vi "X Listbox Facade.vi"(0 "Data In":T4, 2 "Display State In":T2, 3 "Container State":T3) -> (6 "Data Out":T4, 7 "Display State Out":T2, 8 "Action":T1)   [LabVIEW 2011, in "X Listbox-Solution.xctl"]
doc: "This is the facade for the X Listbox. Details about implementation can be found in the course manual.\n\nAAL 9/09"
uses:
  X Listbox-Solution.xctl
  X Listbox Data.ctl
  <vilib>/_xctls/Container State.ctl
  X Listbox State.ctl
  <vilib>/_xctls/Action.ctl
  <vilib>/_xctls/XControlSupport.lvlib
panel:
  in  "True Boolean":bool=TRUE
  in  "False Boolean":bool
  in  "Listbox":i32(listbox)
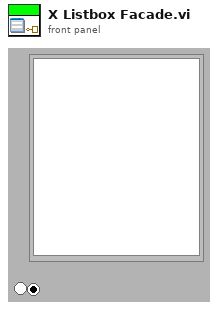
[diagram p1: front panel]
types:
  T1 = typedef "XControlSupport.lvlib/Action.ctl" = cluster{"Data Changed?":bool, "State Changed?":bool, "Action Name":string}
  T2 = typedef "X Listbox-Solution.xctl/X Listbox State.ctl" = cluster{"# Items":i32, "Names":string[]}
  T3 = typedef "XControlSupport.lvlib/Container State.ctl" = cluster{"Indicator?":bool, "Run Mode?":bool, " Refnum":refnum<vi>}
  T4 = typedef "X Listbox-Solution.xctl/X Listbox Data.ctl" = string
  T5 = typedef "imagedata.ctl" = cluster{"image type":i32, "image depth":i32, "image":u8[], "mask":u8[], "colors":u32[], "Rectangle":cluster{"left":i16, "top":i16, "right":i16, "bottom":i16}}
  T6 = typedef "LVPoint32TypeDef.ctl" = cluster{"Horizontal":i32, "Vertical":i32}
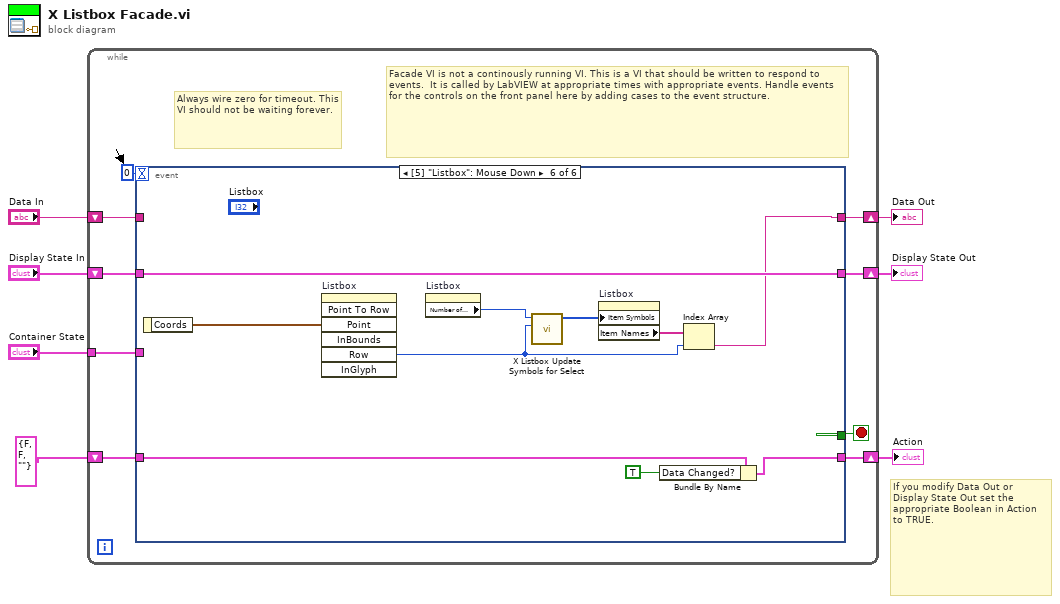
[diagram p0: block diagram]
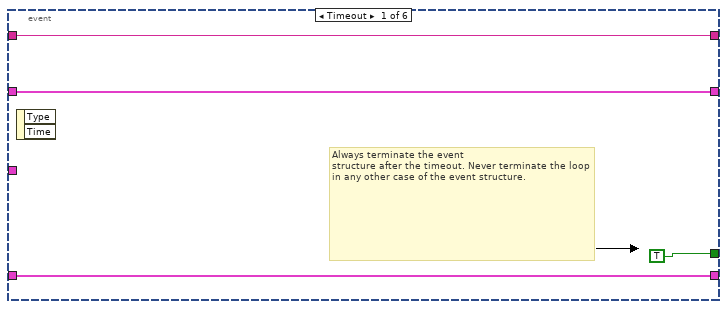
[diagram p2: hidden frame]
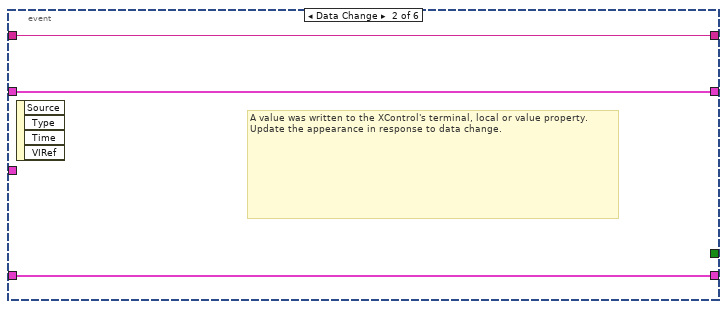
[diagram p3: hidden frame]
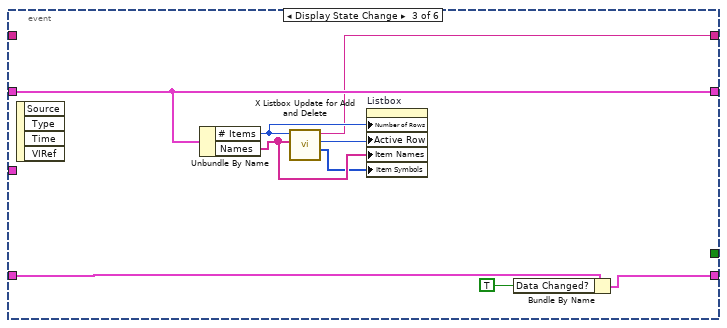
[diagram p4: hidden frame]
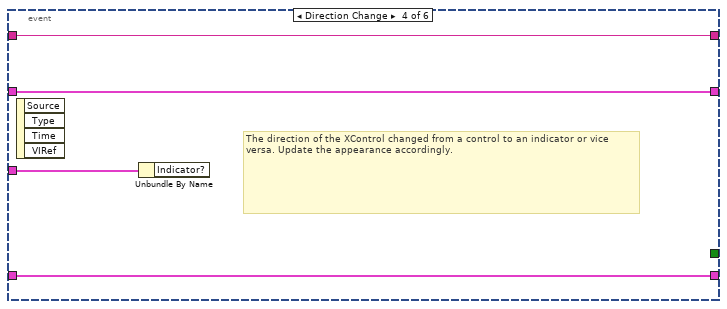
[diagram p5: hidden frame]
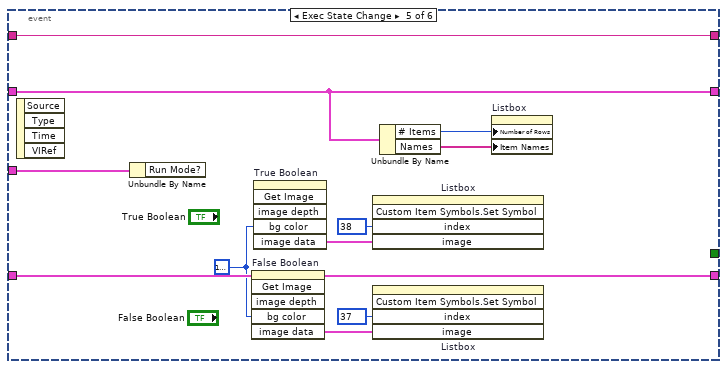
[diagram p6: hidden frame]
diagram:
  # "If you modify Data Out or\nDisplay State Out set the\nappropriate Boolean in Action\nto TRUE."
  n1 = while {
    shift-right: [w15] -> w4
    shift-left: "Display State In" -> [w16]
    tunnel: "Container State" -> [w12]
    shift-right: [w10] -> w7
    shift-left: "Data In" -> [w11]
    shift-right: [w8] -> w2
    shift-left: T1 {"Data Changed?"=FALSE, "State Changed?"=FALSE, "Action Name"=""} ("Action") -> [w9]
    stop <- w14 stop-if-true
    # "Facade VI is not a continously running VI. This is a VI that should be written to respond to events.  It is called by LabVIEW at appropriate times with appropriate events. Handle events for the controls on the front panel here by adding cases to the event structure."
    # "Always wire zero for timeout. This\nVI should not be waiting forever."
    n2 = event shown="[5] \"Listbox\": Mouse Down" {
      selector: _ -> [_ _ _ _ _ _]
      dyn-events: _ -> [_ _ _ _ _ _]
      timeout: 0 -> [_ _ _ _ _ _]
      tunnel: w16 -> [w18 w22 w32 w35 w44 w56]
      tunnel: [w18 w22 w32 w35 w44 w56] -> w15
      tunnel: [TRUE _ _ _ _ _] -> w14
      tunnel: w12 -> [_ _ _ w36 w47 _]
      tunnel: w11 -> [w17 w23 _ w34 w46 _]
      tunnel: [w17 w23 w30 w34 w46 w51] -> w10
      tunnel: [w19 w21 w25 w33 w45 w49] -> w8
      tunnel: w9 -> [w19 w21 w26 w33 w45 w50]
      event Timeout {
        # "Always terminate the event\nstructure after the timeout. Never terminate the loop in any other case of the event structure."
        n3 = event-data() -> ()  [unwired: 1 in, 2 out]
      }
      event Data Change {
        # "A value was written to the XControl's terminal, local or value property.\nUpdate the appearance in response to data change."
        n4 = event-data() -> ()  [unwired: 1 in, 4 out]
      }
      event Display State Change {
        n5 = event-data() -> ()  [unwired: 1 in, 4 out]
        n6 = Unbundle By Name(w32) -> ("# Items"=w31:i32, "Names"=w28:string[])
        n7 = call "X Listbox Update for Add and Delete.vi"("Names"=w28, "# Items"=w31) -> ("Item Symbols"=w27:i32[], "Active Row"=w29:i32, "Name"=w30:string)  [unwired: 7 in]
        n8 = property on="Listbox" class="LstBox (strict)"("Number of Rows"=w31, "Active Row"=w29, "Item Names"=w28, "Item Symbols"=w27) -> ()  [unwired: 2 in, 2 out]
        n9 = Bundle By Name(cluster=w26, "Data Changed?"=TRUE) -> (w25:T1)
      }
      event Direction Change {
        # "The direction of the XControl changed from a control to an indicator or vice versa. Update the appearance accordingly."
        n10 = event-data() -> ()  [unwired: 1 in, 4 out]
        n11 = Unbundle By Name(w36) -> ()  [unwired: 1 out]
      }
      event Exec State Change {
        w40 = u32 16777226
        n12 = event-data() -> ()  [unwired: 1 in, 4 out]
        n13 = Unbundle By Name(w47) -> ()  [unwired: 1 out]
        n14 = invoke on="False Boolean" class="Bool (strict)" method="Get Image"("bg color"=w40) -> ("image data"=w39:T5)  [unwired: 5 in, 5 out]
        n15 = invoke on="True Boolean" class="Bool (strict)" method="Get Image"("bg color"=w40) -> ("image data"=w38:T5)  [unwired: 5 in, 5 out]
        n16 = invoke on="Listbox" class="LstBox (strict)" method="Custom Item Symbols.Set Symbol"("index"=38, "image"=w38) -> ()  [unwired: 3 in, 5 out]
        n17 = invoke on="Listbox" class="LstBox (strict)" method="Custom Item Symbols.Set Symbol"("index"=37, "image"=w39) -> ()  [unwired: 3 in, 5 out]
        n18 = Unbundle By Name(w44) -> ("# Items"=w43:i32, "Names"=w42:string[])
        n19 = property on="Listbox" class="LstBox (strict)"("Number of Rows"=w43, "Item Names"=w42) -> ()  [unwired: 2 in, 2 out]
      }
      event "Listbox": Mouse Down {
        n20 = event-data() -> ("Coords"=w57:T6)  [unwired: 1 in]
        n21 = invoke on="Listbox" class="LstBox (strict)" method="Point To Row"("Point"=w57) -> ("Row"=w52:i32)  [unwired: 6 in, 6 out]
        n22 = property on="Listbox" class="LstBox (strict)"() -> ("Number of Rows"=w55:u32)  [unwired: 2 in, 2 out]
        n23 = call "X Listbox Update Symbols for Select.vi"("Selected Row"=w52, "Number of Rows"=w55) -> ("Item Symbols"=w54:i32[])  [unwired: 9 in]
        n24 = property on="Listbox" class="LstBox (strict)"("Item Symbols"=w54) -> ("Item Names"=w53:string[])  [unwired: 2 in, 2 out]
        n25 = Bundle By Name(cluster=w50, "Data Changed?"=TRUE) -> (w49:T1)
        n26 = Index Array(array=w53, index=w52) -> (element=w51:string)
      }
    }
  }
  "Display State Out" <- w4
  "Data Out" <- w7
  "Action" <- w2
